vi "BinFFT.vi"(6 "Cal Spectrum":cdb[](array[numeric]) format="%.2f", 8 "RF Data Line":dbl[](array[numeric]) format="%.2f", 9 "Tranducer Info":T1 {"start freq" format="%.2f"; "center freq" format="%.2f"; "bandwidth" format="%.2f"}, 10 "A/D info":T2, 11 "Number of bins":i32=3) -> (2 "bin envelopes":dbl[][](graph), 3 "Envelope of\nOutput bins":dbl[](array[numeric]) format="%.2f")   [LabVIEW 2022 SP3]
uses:
  <vilib>/Analysis/baseanly.llb/Mean (DBL).vi
  <vilib>/Analysis/2dsp.llb/Real FFT.vi
  <vilib>/Analysis/4window.llb/Hamming Window (DBL).vi
  <vilib>/Analysis/2dsp.llb/Inverse Complex FFT.vi
  <vilib>/Analysis/4window.llb/AllCosWindow (DBL).vi
  <vilib>/Analysis/NI_AALPro.lvlib
  <vilib>/Analysis/NI_AALBase.lvlib
panel:
  out "rf spectrum":dbl[](graph)
  out "bins in time":dbl[][](graph)
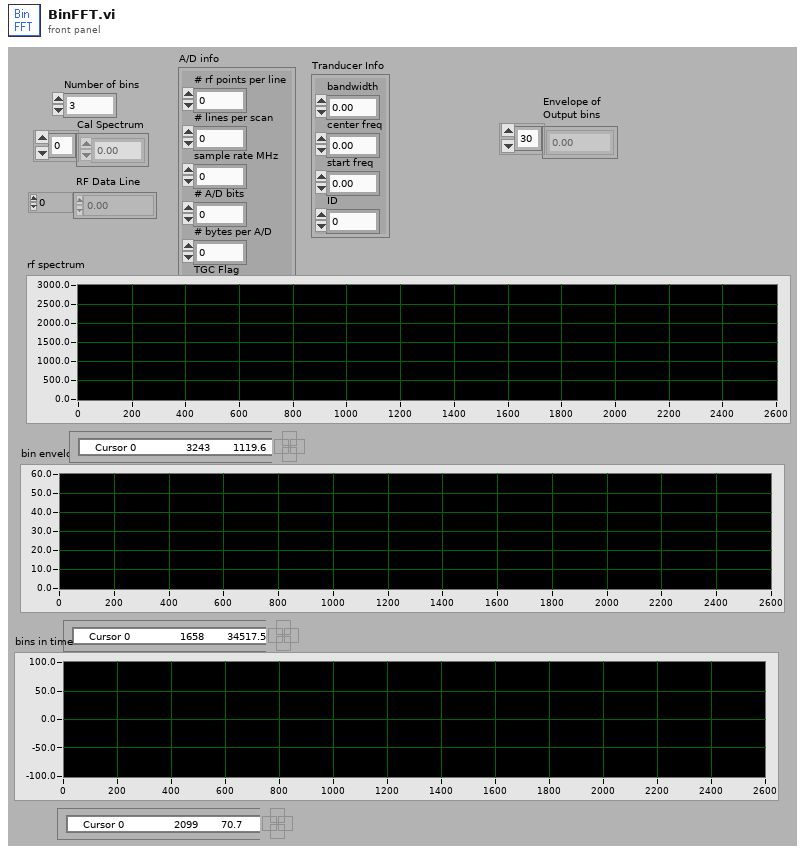
[diagram p1: front panel]
types:
  T1 = cluster{"bandwidth":sgl, "center freq":sgl, "start freq":sgl, "ID":i32}
  T2 = cluster{"# rf points per line":u16, "# lines per scan":u16, "sample rate MHz":u16, "# A/D bits":i16, "# bytes per A/D":u16, "TGC Flag":u16, "A/D Type":string}
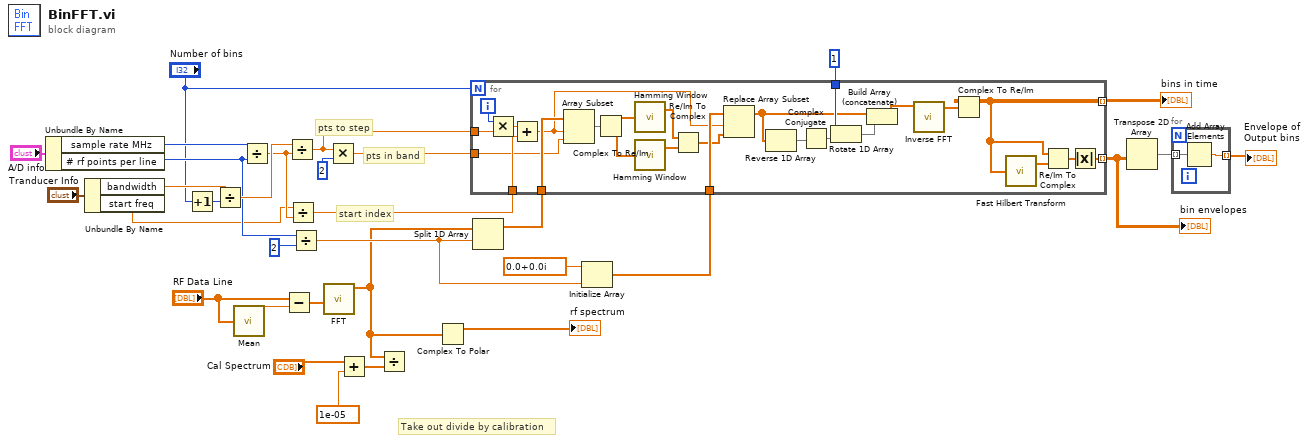
[diagram p0: block diagram]
diagram:
  # "Take out divide by calibration"
  # "pts to step"
  # "pts in band"
  # "start index"
  n1 = Unbundle By Name("A/D info") -> ("sample rate MHz"=w31:u16, "# rf points per line"=w26:u16)
  n2 = Unbundle By Name("Tranducer Info") -> ("bandwidth"=w32:sgl, "start freq"=w19:sgl)
  n3 = Increment(x="Number of bins") -> (x+1=w17:i32)
  n4 = Divide(x=w32, y=w17) -> (x/y=w30:sgl)
  n5 = call-poly <vilib>:"Mean.vi"("X"="RF Data Line") -> ("mean"=w12:dbl)  [unwired: 1 out]
  n6 = Divide(x=w31, y=w26) -> (x/y=w27:dbl)
  n7 = Subtract(x="RF Data Line", y=w12) -> (x-y=w11:dbl[])
  n8 = Divide(x=w30, y=w27) -> (x/y=w21:dbl)
  n9 = Divide(x=w19, y=w27) -> (x/y=w23:dbl)
  n10 = Divide(x=w26, y=2) -> (x/y=w20:dbl)
  n11 = call-poly <vilib>:"FFT.vi"("X"=w11) -> ("FFT {X}"=w4:cdb[])  [unwired: 2 in, 8 out]
  n12 = Multiply(x=w21, y=2) -> (x*y=w22:dbl)
  n13 = Add(x="Cal Spectrum", y=1e-05) -> (x+y=w6:cdb[])
  n14 = Divide(x=w4, y=w6) -> ()  [unwired: 1 out]
  n15 = Complex To Polar(r * e^(i*theta)=w4) -> (r=→"rf spectrum":dbl[])  [unwired: 1 out]
  n16 = Split 1D Array(array=w4, index=w20) -> (first subarray=w10:cdb[])  [unwired: 1 out]
  n17 = Initialize Array(cdb 0.0+0.0i, w20) -> (w24:cdb[])
  n18 = for {
    N: "Number of bins" -> [_]
    tunnel: w10 -> [w57]
    tunnel: w24 -> [w55]
    tunnel: [w36] -> w7 mode=indexing
    tunnel: w23 -> [w46]
    tunnel: w22 -> [w34]
    tunnel: w21 -> [w45]
    tunnel: 1 -> [w43]
    tunnel: [w35] -> w2 mode=indexing
    i -> [w56]
    n19 = Multiply(x=w56, y=w45) -> (x*y=w47:dbl)
    n20 = Add(x=w47, y=w46) -> (x+y=w33:dbl)
    n21 = Array Subset(array=w57, index=w33, length=w34) -> (w54:cdb[])
    n22 = Complex To Re/Im(x + iy=w54) -> (x=w53:dbl[], y=w52:dbl[])
    n23 = call-poly <vilib>:"Hamming Window.vi"("X"=w53) -> ("Windowed X"=w50:dbl[])  [unwired: 1 out]
    n24 = call-poly <vilib>:"Hamming Window.vi"("X"=w52) -> ("Windowed X"=w51:dbl[])  [unwired: 1 out]
    n25 = Re/Im To Complex(1:w51, 2:w50) -> (0:w49:cdb[])
    n26 = Replace Array Subset(array=w55, new element=w49, index=w33) -> (w41:cdb[])
    n27 = Reverse 1D Array(array=w41) -> (reversed array=w48:cdb[])
    n28 = Complex Conjugate(1:w48) -> (0:w44:cdb[])
    n29 = Rotate 1D Array(1:w44, 2:w43) -> (0:w40:cdb[])
    n30 = Build Array (concatenate)(w41, w40) -> (w42:cdb[])
    n31 = call-poly <vilib>:"Inverse FFT.vi"("FFT {X}"=w42) -> ("X"=w37:cdb[])  [unwired: 1 in, 9 out]
    n32 = Complex To Re/Im(x + iy=w37) -> (x=w36:dbl[])  [unwired: 1 out]
    n33 = call <vilib>:"Fast Hilbert Transform.vi"("X"=w36) -> ("Hilbert{X}"=w38:dbl[])  [unwired: 1 out]
    n34 = Re/Im To Complex(1:w38, 2:w36) -> (0:w39:cdb[])
    n35 = Absolute Value(x=w39) -> (abs(x)=w35:dbl[])
  }
  "bin envelopes" <- w2
  "bins in time" <- w7
  n36 = Transpose 2D Array(2D array=w2) -> (transposed array=w3:dbl[][])
  n37 = for {
    tunnel: w3 -> [w59] mode=indexing
    tunnel: [w58] -> w1 mode=indexing
    n38 = Add Array Elements(numeric array=w59) -> (sum=w58:dbl)
  }
  "Envelope of\nOutput bins" <- w1
